vi "File_Settings Requested Path.vi"() -> (3 "Requested Path":path)   [LabVIEW 2021]
uses:
  vi.lib/LabVIEW Icon API/lv_icon/Controls/Pathes.ctl
  vi.lib/LabVIEW Icon API/lv_icon/lv_icon.lvlib
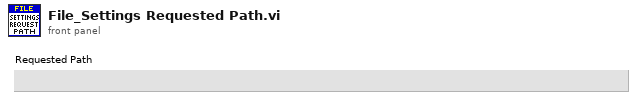
[diagram p1: front panel]
types:
  T1 = typedef "Pathes.ctl" = enum16{"Root Path", "Icon Templates", "Icon Templates VI", "Icon Templates Lib", "Glyphs"}
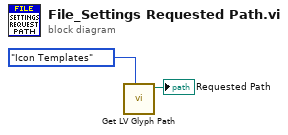
[diagram p0: block diagram]
diagram:
  n1 = call "Get LV Glyph Path.vi"("Path"=Pathes."Icon Templates") -> ("Requested Path"=→"Requested Path":path)  [unwired: 2 in, 8 out]
